vi "add modification.vi"(6 "parameters":variant[](array[variant]), 8 "error in":errorcluster, 9 "exclusions":string[](array[string]), 10 "VI Refnum":refnum<vi>, 11 "vi modification tool in":refnum<class "vi modification tool.lvclass">) -> (0 "error out":errorcluster, 3 "vi modification tool out":refnum<class "vi modification tool.lvclass">)   [LabVIEW 2013, in "vi modification tool.lvclass"]
uses:
  vi modification tool.lvclass
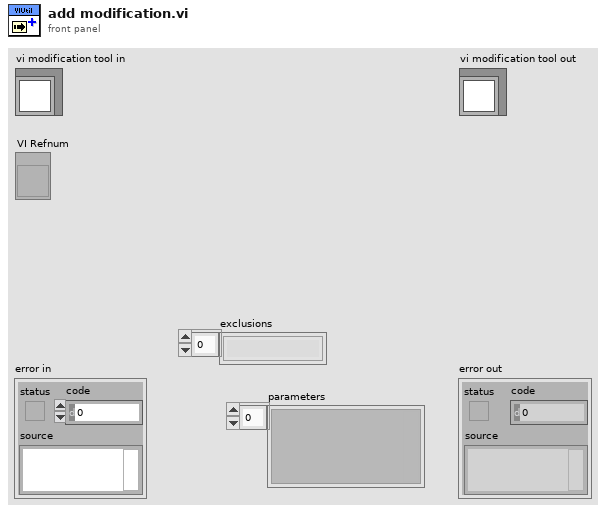
[diagram p1: front panel]
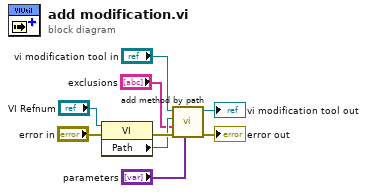
[diagram p0: block diagram]
diagram:
  n1 = property class="VI"(reference="VI Refnum", error in="error in") -> (error out=w4:errorcluster, "Path"=w3:path)  [unwired: 1 out]
  n2 = call "add method by path.vi"("parameters"="parameters", "error in"=w4, "exclusions"="exclusions", "Path"=w3, "vi modification tool in"="vi modification tool in") -> ("error out"=→"error out":errorcluster, "vi modification tool out"=→"vi modification tool out":refnum<class "vi modification tool.lvclass">)  [unwired: 5 in]
